vi "NewLot.vi"(5 "Enum":enum16{"LOAD", "NEW"}(ring)=enum."NEW", 7 "Create Entry?":bool, 8 "error in (no error)":errorcluster, 9 "Test":string, 10 "Wafer ID":string, 11 "FrontPanelData in":refnum<class "EpiWrapper.lvclass">) -> (0 "error out":errorcluster, 2 "DB Message":string, 3 "FrontPanelData out":refnum<class "EpiWrapper.lvclass">)   [LabVIEW 2012, in "EpiWrapper.lvclass"]
uses:
  Classes/EpiWrapper.lvclass
  Classes/EpiWrapper.lvclass/EpiWrapper.ctl
  Classes/LotData.lvclass
  Controls/UserInput.ctl
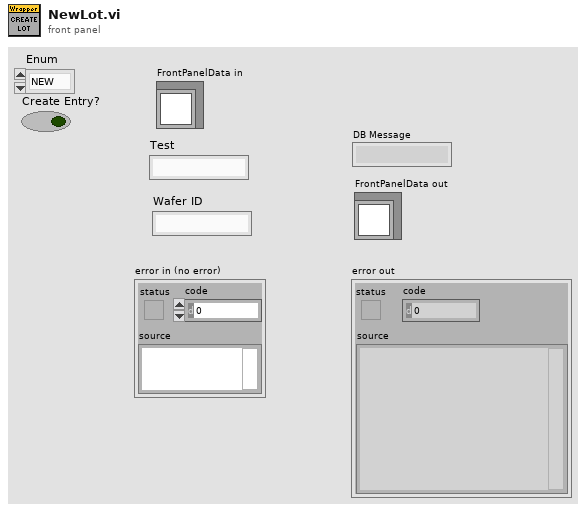
[diagram p1: front panel]
types:
  T1 = typedef "UserInput.ctl" = cluster{"Wafer ID":string, "Test":string, "New":bool, "Save":bool, "Load":bool, "Cancel":bool}
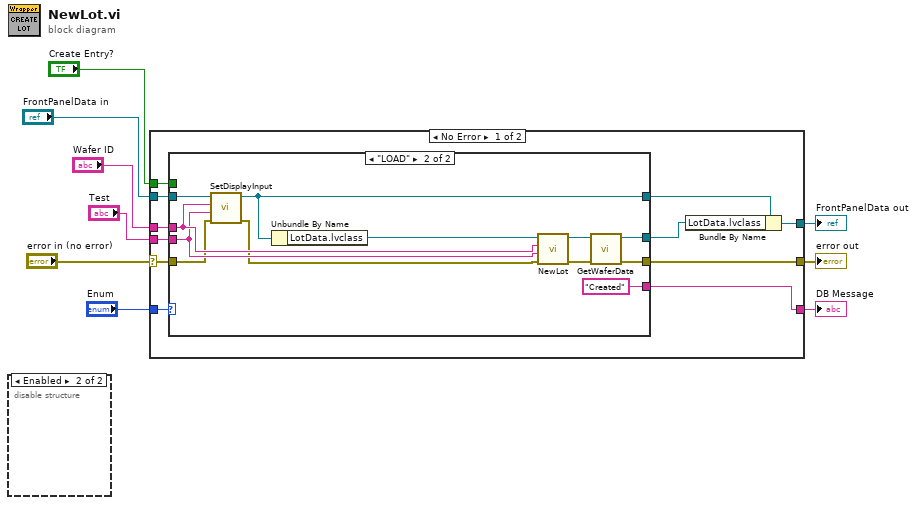
[diagram p0: block diagram]
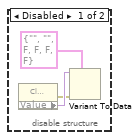
[diagram p2: hidden frame]
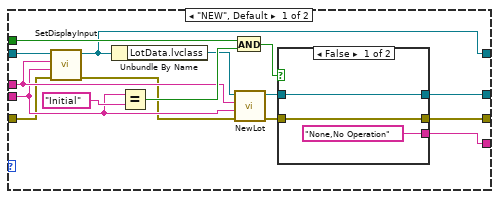
[diagram p3: hidden frame]
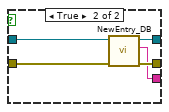
[diagram p4: hidden frame]
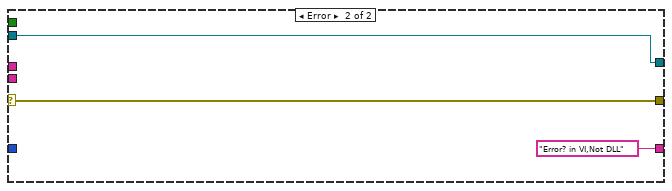
[diagram p5: hidden frame]
diagram:
  n1 = disable-structure shown="Enabled" {
    frame Disabled {
      n2 = property class="Clust"() -> (error out=w11:errorcluster, "Value"=w12:variant)  [unwired: 2 in, 1 out]
      n3 = Variant To Data(error in=w11, type=T1 {"Wafer ID"="", "Test"="", "New"=FALSE, "Save"=FALSE, "Load"=FALSE, "Cancel"=FALSE} ("Cluster 2"), Variant=w12) -> ()  [unwired: 2 out]
    }
    frame Enabled {
    }
  }
  n4 = case shown="No Error" "error in (no error)" {
    selector: "error in (no error)" -> [w22 w62]
    tunnel: [w19 w62] -> w8
    tunnel: [w21 w61] -> w6
    tunnel: "FrontPanelData in" -> [w23 w61]
    tunnel: [w15 "Error? in VI,Not DLL" ("DB Message")] -> w5
    tunnel: "Wafer ID" -> [w14 _]
    tunnel: "Test" -> [w13 _]
    tunnel: "Enum" -> [w17 _]
    tunnel: "Create Entry?" -> [w18 _]
    frame No Error {
      n5 = case shown="\"LOAD\"" w17 {
        tunnel: w23 -> [w30 w54]
        tunnel: w22 -> [w25 w49]
        tunnel: [w38 w57] -> w20
        tunnel: [w36 w56] -> w19
        tunnel: w18 -> [w34 _]
        tunnel: [w29 w52] -> w16
        tunnel: [w32 "Created" ("NewWaferEntry")] -> w15
        tunnel: w14 -> [w27 w51]
        tunnel: w13 -> [w26 w50]
        frame "NEW", Default {
          n6 = call-dynamic "SetDisplayInput.vi"("error in (no error)"=w25, "Test"=w26, "Wafer ID"=w27, "EpiWrapper in"=w30) -> ("error out"=w24:errorcluster, "EpiWrapper out"=w29:refnum<class "EpiWrapper.lvclass">)  [unwired: 6 in]
          n7 = Unbundle By Name(w29) -> ("LotData.lvclass"=w28:refnum<class "LotData.lvclass">)
          n8 = Equal?(x=w26, y="Initial" ("Test")) -> (x = y?=w35:bool)
          n9 = And(x=w34, y=w35) -> (x .and. y?=w33:bool)
          n10 = call "NewLot.vi"("error in (no error)"=w24, "Type"=w26, "Wafer ID"=w27, "LotData in"=w28) -> ("error out"=w37:errorcluster, "LotData out"=w39:refnum<class "LotData.lvclass">)  [unwired: 6 in]
          n11 = case shown="False" w33 {
            tunnel: ["None,No Operation" ("DB Message") w43] -> w32
            tunnel: w39 -> [w41 w47]
            tunnel: [w41 w46] -> w38
            tunnel: w37 -> [w40 w45]
            tunnel: [w40 w44] -> w36
            frame False {
            }
            frame True {
              n12 = call-dynamic "NewEntry_DB.vi"("error in (no error)"=w45, "LotData in"=w47) -> ("error out"=w44:errorcluster, "NewWaferEntry"=w43:string, "LotData out"=w46:refnum<class "LotData.lvclass">)  [unwired: 7 in]
            }
          }
        }
        frame "LOAD" {
          n13 = call-dynamic "SetDisplayInput.vi"("error in (no error)"=w49, "Test"=w50, "Wafer ID"=w51, "EpiWrapper in"=w54) -> ("error out"=w48:errorcluster, "EpiWrapper out"=w52:refnum<class "EpiWrapper.lvclass">)  [unwired: 6 in]
          n14 = Unbundle By Name(w52) -> ("LotData.lvclass"=w53:refnum<class "LotData.lvclass">)
          n15 = call "NewLot.vi"("error in (no error)"=w48, "Type"=w50, "Wafer ID"=w51, "LotData in"=w53) -> ("error out"=w58:errorcluster, "LotData out"=w59:refnum<class "LotData.lvclass">)  [unwired: 6 in]
          n16 = call-dynamic "GetWaferData.vi"("error in (no error)"=w58, "LotData in"=w59) -> ("error out"=w56:errorcluster, "LotData out"=w57:refnum<class "LotData.lvclass">)  [unwired: 8 in]
        }
      }
      n17 = Bundle By Name(cluster=w16, "LotData.lvclass"=w20) -> (w21:refnum<class "EpiWrapper.lvclass">)
    }
    frame Error {
    }
  }
  "error out" <- w8
  "FrontPanelData out" <- w6
  "DB Message" <- w5
